vi "Analyze DC Voltage Measurements.vi"(8 "error in":errorcluster, 10 "Volatge Waveforms":waveform(dbl)[](array[waveform])) -> (0 "error out":errorcluster, 1 "RMS values":dbl[](array[numeric]), 2 "DC values":dbl[](array[numeric]))   [LabVIEW 2024, in "NIDmmDCRmsVoltage.lvlib"]
uses:
  NIDmmDCRmsVoltage.lvlib
  <vilib>/measure/NI_MAPro.lvlib
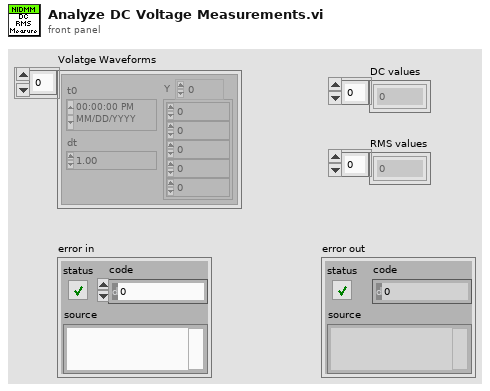
[diagram p1: front panel]
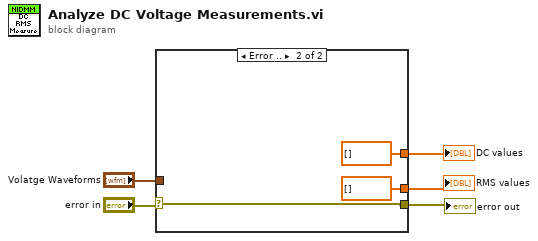
[diagram p0: block diagram]
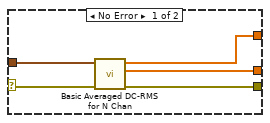
[diagram p2: hidden frame]
diagram:
  n1 = case shown="Error .." "error in" {
    selector: "error in" -> [w9 w13]
    tunnel: [w10 w13] -> w4
    tunnel: "Volatge Waveforms" -> [w8 _]
    tunnel: [w7 dbl[] [] ("RMS values")] -> w2
    tunnel: [w6 dbl[] [] ("DC values")] -> w3
    frame No Error {
      n2 = call <vilib>:"Basic Averaged DC-RMS for N Chan.vi"("error in (no error)"=w9, "signals in"=w8) -> ("error out"=w10:errorcluster, "RMS values"=w7:dbl[], "DC values"=w6:dbl[])  [unwired: 6 in, 1 out]
    }
    frame Error {
    }
  }
  "DC values" <- w3
  "RMS values" <- w2
  "error out" <- w4
